vi "Set Node ID.vi"(8 "error in (no error)":errorcluster, 10 "Node ID":u32, 11 "Node in":refnum<class "Node Config.lvclass">) -> (0 "error out":errorcluster, 3 "Node out":refnum<class "Node Config.lvclass">)   [LabVIEW 2020, in "VolatusConfig.lvlib" / "Node Config.lvclass"]
uses:
  Node Config.lvclass
  C:/dev/lv20CE/relink/lv-volatus/VolatusConfig/VolatusConfigElement/VolatusConfigElement.lvclass
  lv-cdm/CDM-Config/Value Type.ctl
  VolatusConfigElement/VolatusConfigElement.lvclass/VolatusConfigElement.ctl
  lv-cdm/CDM-Config/Config Element/Write Variant Value.vi
  Node Config.lvclass/Node Config.ctl
  lv-cdm/CDM-Config/Config Element/Config Element.lvclass
  VolatusConfigElement/VolatusConfigElement.lvclass
  lv-cdm/CDM-Config/CDM-Config.lvlib
  C:/dev/lv20CE/relink/lv-volatus/VolatusConfig/Node/Node Config.lvclass
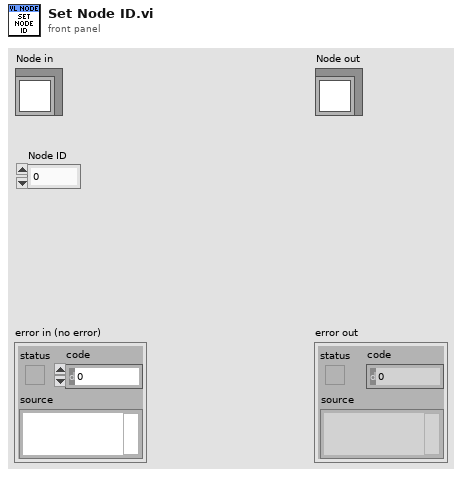
[diagram p1: front panel]
types:
  T1 = typedef "CDM-Config.lvlib/Value Type.ctl" = enum16{"String", "Number", "Bool", "Object", "Array"}
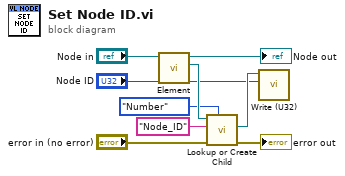
[diagram p0: block diagram]
diagram:
  n1 = call "Element.vi"("VolatusConfigElement in"="Node in") -> ("Element"=w7:refnum<class "Config Element.lvclass">, "VolatusConfigElement out"=→"Node out":refnum<class "Node Config.lvclass">)  [unwired: 9 in]
  n2 = call "Lookup or Create Child.vi"("Value Type (Object)"=Value_Type."Number" ("Value Type (String)"), "error in (no error)"="error in (no error)", "Name"="Node_ID", "Config Element in"=w7) -> ("error out"=→"error out":errorcluster, "Child"=w2:refnum<class "Config Element.lvclass">)  [unwired: 4 in, 2 out]
  n3 = call "Write (U32).vi"("U32 Value"="Node ID", "Config Element in"=w2) -> ()  [unwired: 8 in, 2 out]
